vi "Error Message.vi"(0 "VISA Resource Name":refnum<visa-resource-name>, 5 "Type of Dialog (OK msg:1)":u16(ring)=1 items=["No Dialog", "OK Message", "Continue or Stop Message"], 11 "error in (no error)":errorcluster {"code" format="%.0x"}) -> (3 "Status":bool, 4 "VISA Resource Name Out":refnum<visa-resource-name>, 8 "Error Code (0)":i32, 10 "Error Message (empty)":string, 15 "error out":errorcluster {"code" format="%.0x"})   [LabVIEW 2020, in "Olympus IX BX Series.lvlib"]
doc: "Contains all the instrument-specific error codes and descriptions."
uses:
  Olympus IX BX Series.lvlib
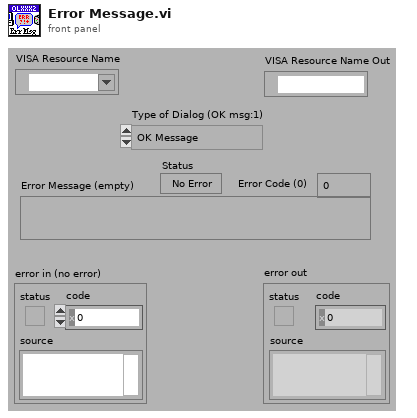
[diagram p1: front panel]
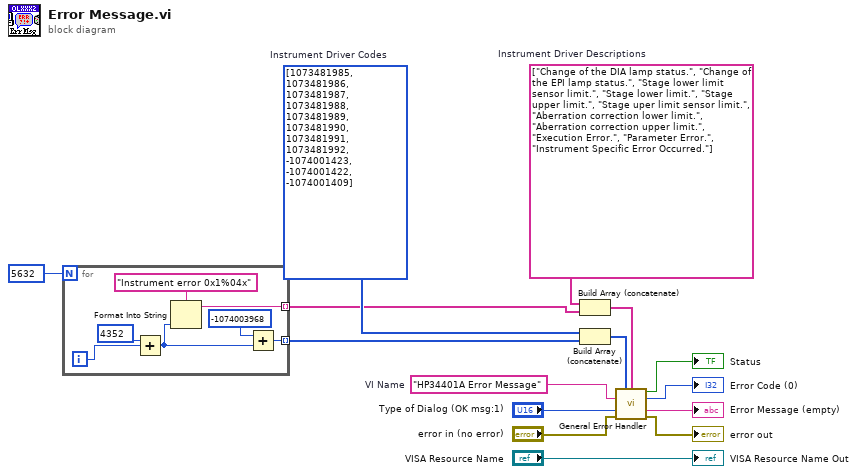
[diagram p0: block diagram]
diagram:
  w5 = string[] ["Change of the DIA lamp status.", "Change of the EPI lamp status.", "Stage lower limit sensor limit.", "Stage lower limit.", "Stage upper limit.", "Stage uper limit sensor limit.", "Aberration correction lower limit.", "Aberration correction upper limit.", "Execution Error.", "Parameter Error.", "Instrument Specific Error Occurred."]  # Instrument Driver Descriptions
  w4 = i32[] [1073481985, 1073481986, 1073481987, 1073481988, 1073481989, 1073481990, 1073481991, 1073481992, -1074001423, -1074001422, -1074001409]  # Instrument Driver Codes
  w12 = "HP34401A Error Message"  # VI Name
  n1 = for {
    N: 5632 -> [_]
    tunnel: [w20] -> w3 mode=indexing
    tunnel: [w19] -> w2 mode=indexing
    i -> [w17]
    n2 = Add(x=4352, y=w17) -> (x+y=w16:i32)
    n3 = Format Into String(format string="Instrument error 0x1%04x", w16) -> (resulting string=w19:string)  [unwired: 2 in, 1 out]
    n4 = Add(x=-1074003968, y=w16) -> (x+y=w20:i32)
  }
  n5 = Build Array (concatenate)(w5, w2) -> (w7:string[])
  n6 = Build Array (concatenate)(w4, w3) -> (w6:i32[])
  n7 = call <vilib>:"General Error Handler.vi"("[user-defined codes]"=w6, "[user-defined descriptions]"=w7, "[error source] (\" \")"=w12, "type of dialog (OK msg:1)"="Type of Dialog (OK msg:1)", "error in (no error)"="error in (no error)") -> ("error?"=→"Status":bool, "code out"=→"Error Code (0)":i32, "message"=→"Error Message (empty)":string, "error out"=→"error out":errorcluster)  [unwired: 6 in, 1 out]
  "VISA Resource Name Out" <- "VISA Resource Name"
